vi "preparePassScore.vi"(8 "error in (no error)":errorcluster, 9 "OffensiveTeam":refnum<class "Ally.lvclass">, 10 "OffensivePlay":T1=enum."PrepareTriplePass", 11 "Play in":refnum<class "Play.lvclass">) -> (0 "error out":errorcluster, 2 "score":dbl, 3 "Play out":refnum<class "Play.lvclass">)   [LabVIEW 2021, in "Play.lvclass"]
uses:
  Play.lvclass
  Ally_class/Ally.lvclass
  Team_class/OffensivePlay.ctl
  Ally_class/Ally.lvclass/Ally.ctl
  Ally_class/Read PreparePassPlaysEnum.vi
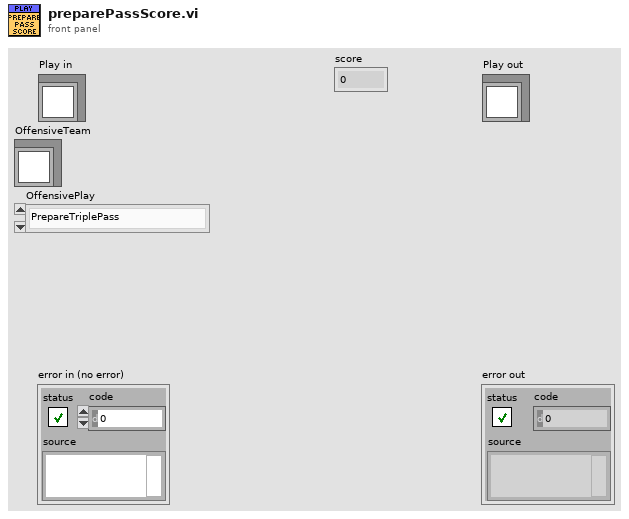
[diagram p1: front panel]
types:
  T1 = typedef "OffensivePlay.ctl" = enum16{"5RobotsPassGamePlay", "5PreparePassGame", "5RobotsKeeperGame", "KeeperPassToStriker", "5RobotsNormalGamePlay", "PrepareKeeperPass", "ACBPass", "ABCPass", "PrepareTriplePass", "TableWithStriker", "TableWith2ndStrikerPlay", "PrepareDoublePass", "PrepareRollToPass", "SimplePass", "PreparePass", "PassToStriker", "BallOutOfField", "PassTo2ndStriker", "StopOffensive", "Prepare Penalty Enemy", "EnemyPossessionAtEnemyField", "EnemyPossesionAtOurField", "TestPlay", "PreparePenaltyAlly", "KickPenaltyAlly", "PrepareKickoffAlly", "PrepareKickoffEnemy", "IndirectEnemy", "DirectEnemy", "PreparePassInGame1", "NormalGame", "DirectKick", "Pass", "Halt", "Timeout", "PassPlay", "PenaltyEnemy"}
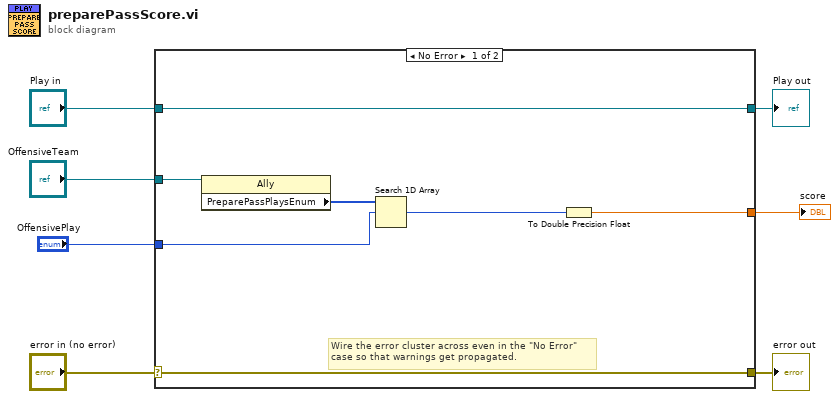
[diagram p0: block diagram]
diagram:
  n1 = case shown="No Error" "error in (no error)" {
    selector: "error in (no error)" -> [w13 w16]
    tunnel: [w13 w16] -> w6
    tunnel: [w14 w15] -> w4
    tunnel: "Play in" -> [w14 w15]
    tunnel: "OffensiveTeam" -> [w12 _]
    tunnel: [w8 _] -> w2
    tunnel: "OffensivePlay" -> [w10 _]
    frame No Error {
      # "Wire the error cluster across even in the \"No Error\"\ncase so that warnings get propagated."
      n2 = property class="Ally"(reference=w12) -> ("PreparePassPlaysEnum"=w11:T1[])  [unwired: 1 in, 2 out]
      n3 = Search 1D Array(1D array=w11, element=w10) -> (index of element=w9:i32)  [unwired: 1 in]
      n4 = To Double Precision Float(number=w9) -> (double precision float=w8:dbl)
    }
    frame Error {
    }
  }
  "error out" <- w6
  "Play out" <- w4
  "score" <- w2
